vi "Primera VI.vi"() -> ()   [LabVIEW 2020]
panel:
  in  "Numeric 2":dbl
  out "Meter":dbl(knob) scale=0.0..10.0
  out "Thermometer":dbl(slide) scale=0.0..100.0
  in  "Numeric":dbl
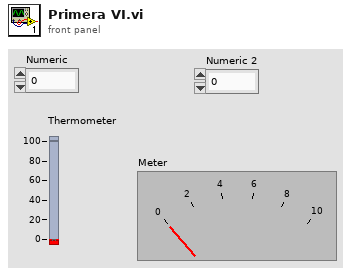
[diagram p1: front panel]
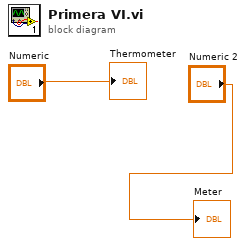
[diagram p0: block diagram]
diagram:
  "Thermometer" <- "Numeric"
  "Meter" <- "Numeric 2"
